vi "closures tests 1.vi"   [LabVIEW 2018]
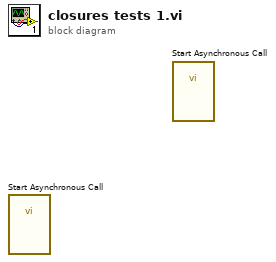
[diagram p0: block diagram]
diagram:
  n1 = call-by-ref "Start Asynchronous Call"() -> ()  [unwired: 11 in, 5 out]
  n2 = call-by-ref "Start Asynchronous Call"() -> ()  [unwired: 14 in, 2 out]
